vi "Pane.vi"(8 "error in":errorcluster, 11 "Gen Refnum":refnum<vi>) -> (0 "error out":errorcluster, 3 "Pane out":refnum<class "Pane.lvclass">)   [LabVIEW 2014, in "Pane.lvclass"]
uses:
  Pane.lvclass
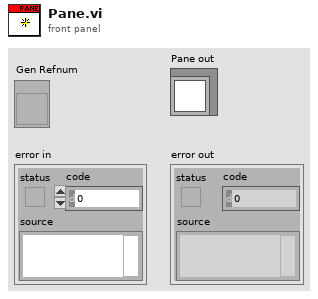
[diagram p1: front panel]
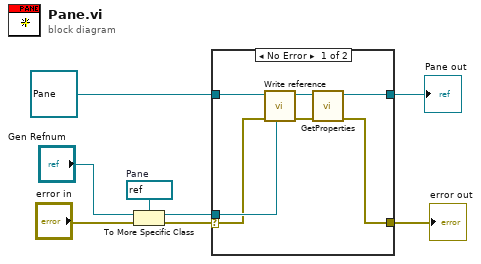
[diagram p0: block diagram]
diagram:
  w5 = refnum<vi> refnum  # Pane
  n1 = To More Specific Class(target class=w5, reference="Gen Refnum", error in="error in") -> (specific class reference=w8:refnum<vi>, error out=w7:errorcluster)
  n2 = case shown="No Error" w7 {
    selector: w7 -> [w12 w17]
    tunnel: refnum<class "Pane.lvclass"> refnum ("Pane in") -> [w15 w16]
    tunnel: w8 -> [w13 _]
    tunnel: [w10 w16] -> w2
    tunnel: [w9 w17] -> w1
    frame No Error {
      n3 = call-dynamic "Write reference.vi"("reference"=w13, "error in"=w12, "GObject in"=w15) -> ("error out"=w11:errorcluster, "GObject out"=w14:refnum<class "Pane.lvclass">)  [unwired: 5 in]
      n4 = call-dynamic "GetProperties.vi"("error in"=w11, "Pane in"=w14) -> ("error out"=w9:errorcluster, "Pane out"=w10:refnum<class "Pane.lvclass">)  [unwired: 8 in]
    }
    frame Error {
    }
  }
  "error out" <- w1
  "Pane out" <- w2
